vi "Plot Data - Configure Plot GUI.vi"(8 "Error In":errorcluster, 11 "Plot Channel Configurations In":T1[](array[typedef])) -> (0 "Error Out":errorcluster, 3 "Plot Channel Configurations Out":T1[](array[typedef]))   [LabVIEW 2017, in "DTacq Plot Display Library.lvlib"]
uses:
  DTacq Plot Display Library.lvlib
  Typedefs/Plot Channel Configruation--Cluster.ctl
  Typedefs/Graphical Interface Commands - Configuration--Enum.ctl
  Network Shared Variables/Typedefs/Shared Variable Properties--Cluster.ctl
  Network Shared Variables/Shared Variables Library.lvlib
panel:
  in  "Paste Button":bool
  in  "Cancel Button":bool
  in  "OK Button":bool
  in  "Plot Colour Box":u32(colorbox)
  in  "Multicolumn Listbox":i32(listbox)
  in  "Descriptive Name":string
  in  "Data Source Dropdown":u16(ring) items=["Carrier1Module1-ACQ425ELF-Channel_01", "Carrier1Module1-ACQ425ELF-Channel_02", "Carrier1Module1-ACQ425ELF-Channel_03", "Carrier1Module1-ACQ425ELF-Channel_04", "Carrier1Module1-ACQ425ELF-Channel_05", "Carrier1Module1-ACQ425ELF-Channel_06", "Carrier1Module1-ACQ425ELF-Channel_07", "Carrier1Module1-ACQ425ELF-Channel_08", "Carrier1Module1-ACQ425ELF-Channel_09", "Carrier1Module1-ACQ425ELF-Channel_10", "Carrier1Module1-ACQ425ELF-Channel_11", "Carrier1Module1-ACQ425ELF-Channel_12", "Carrier1Module1-ACQ425ELF-Channel_13", "Carrier1Module1-ACQ425ELF-Channel_14", "Carrier1Module1-ACQ425ELF-Channel_15", "Carrier1Module1-ACQ425ELF-Channel_16"]
  in  "Remove Button":bool
  in  "Add Button":bool
  # "Data Sources"
  # "Data Source"
  # "Name"
  # "Colour"
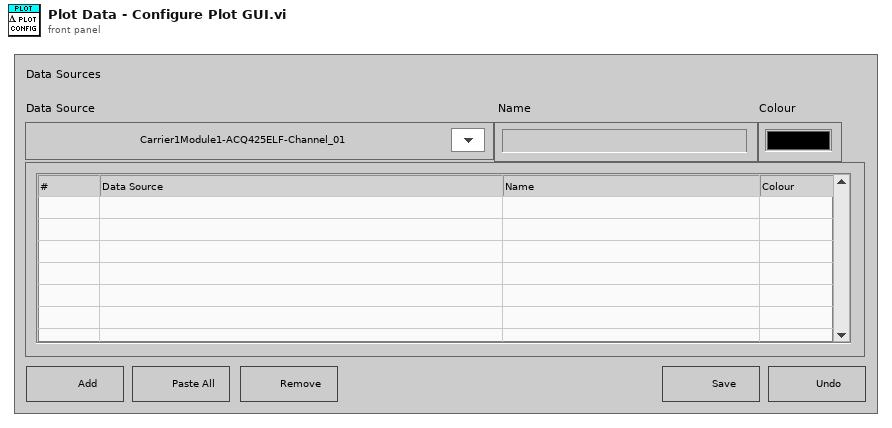
[diagram p1: front panel]
types:
  T1 = typedef "DTacq Plot Display Library.lvlib/Plot Channel Configruation--Cluster.ctl" = cluster{"Shared Variable Reference":refnum<k21>, "Full Variable Name":string, "URL":string, "Descriptive Name":string, "Data Type":variant, "Colour":u32}
  T2 = typedef "Shared Variables Library.lvlib/Shared Variable Properties--Cluster.ctl" = cluster{"Name":string, "URL":string, "Data Type":variant}
  T3 = typedef "DTacq Plot Display Library.lvlib/Graphical Interface Commands - Configuration--Enum.ctl" = enum16{"Cancel and Close", "Paste All", "Restore Previous", "Poll GUI", "Cancel", "Save", "Remove Channel", "Add Channel", "Initialise"}
  T4 = enum32{"Invalid", "Standard", "Closed", "Hidden", "Minimized", "Maximized"}
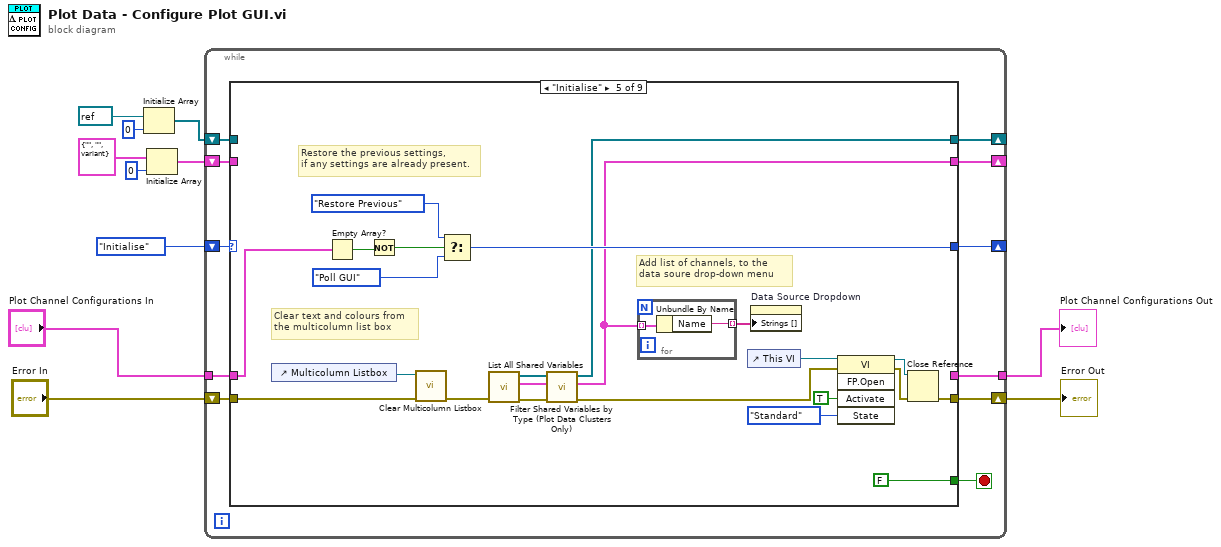
[diagram p0: block diagram]
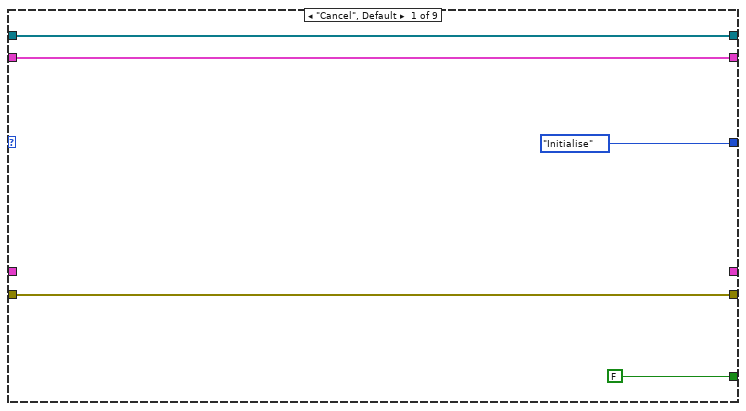
[diagram p2: hidden frame]
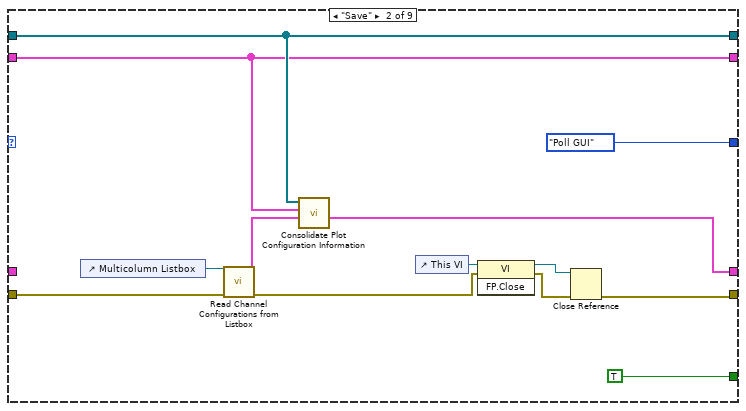
[diagram p3: hidden frame]
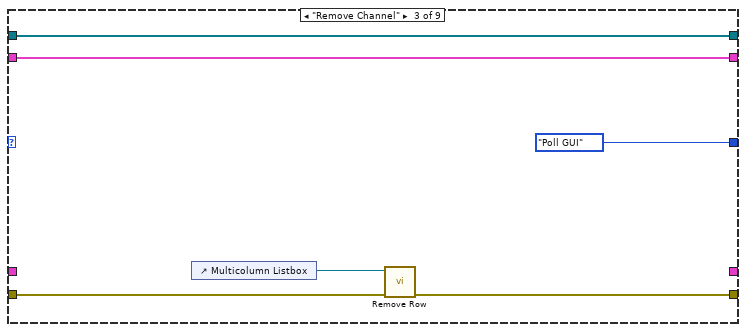
[diagram p4: hidden frame]
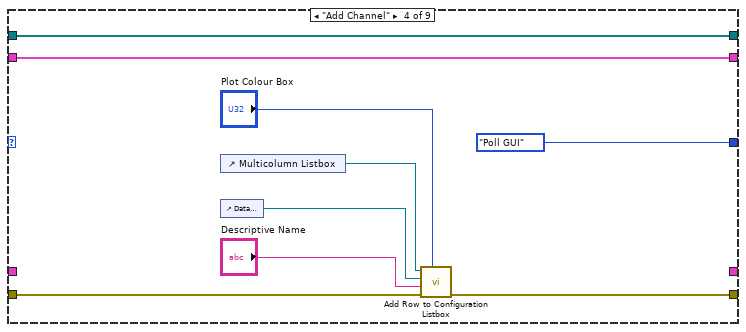
[diagram p5: hidden frame]
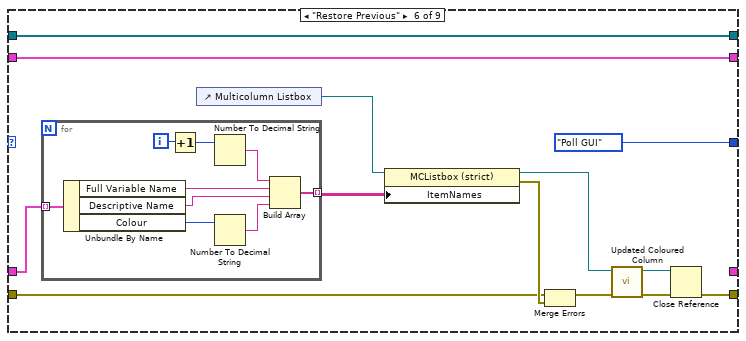
[diagram p6: hidden frame]
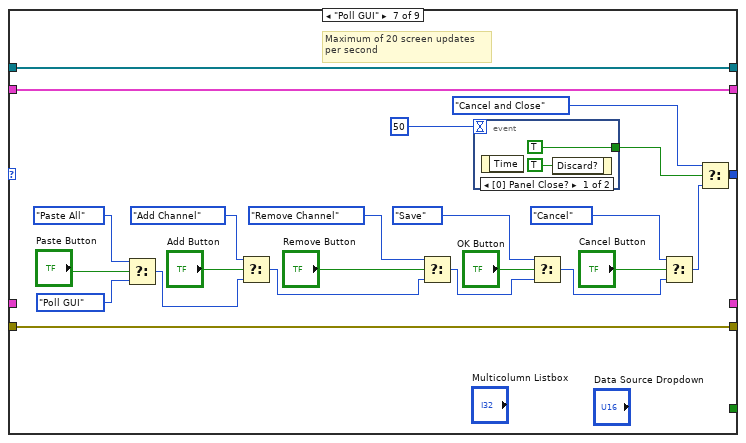
[diagram p7: hidden frame]
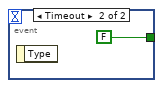
[diagram p8: hidden frame]
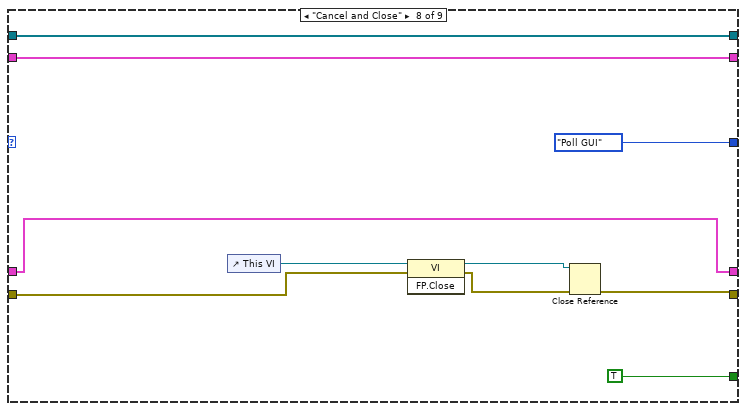
[diagram p9: hidden frame]
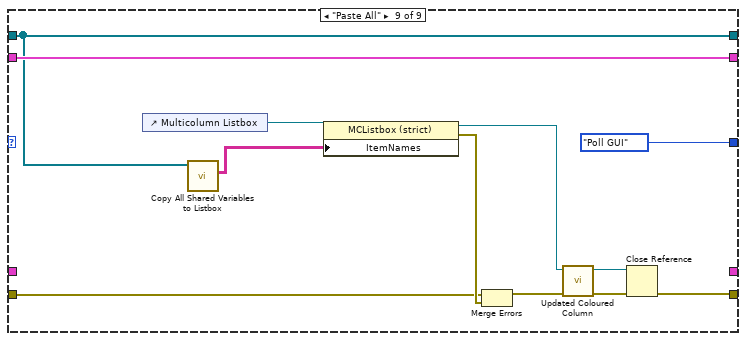
[diagram p10: hidden frame]
diagram:
  n1 = Initialize Array(refnum<k21> refnum, 0 ("dimension size")) -> (w8:refnum<k21>[])
  n2 = Initialize Array(T2 {"Name"="", "URL"="", "Data Type"=variant} ("Shared Variable Data"), 0 ("dimension size")) -> (w5:T2[])
  n3 = while {
    shift-right: [w20] -> w1
    shift-left: "Error In" -> [w21]
    shift-right: [w18] -> _
    shift-left: Graphical_Interface_Commands_-_Configuration--Enum."Initialise" -> [w22]
    shift-right: [w17] -> _
    shift-left: w8 -> [w16]
    shift-right: [w15] -> _
    shift-left: w5 -> [w14]
    tunnel: [w13] -> w4
    tunnel: "Plot Channel Configurations In" -> [w12]
    stop <- w19 stop-if-true
    n4 = case shown="\"Initialise\"" w22 {
      tunnel: w21 -> [w23 w35 w44 w54 w75 w85 w125 w135 w144]
      tunnel: [w23 w28 w43 w49 w70 w87 w125 w134 w140] -> w20
      tunnel: [FALSE TRUE _ _ FALSE _ _ TRUE _] -> w19
      tunnel: [Graphical_Interface_Commands_-_Configuration--Enum."Initialise" Graphical_Interface_Commands_-_Configuration--Enum."Poll GUI" Graphical_Interface_Commands_-_Configuration--Enum."Poll GUI" Graphical_Interface_Commands_-_Configuration--Enum."Poll GUI" w62 Graphical_Interface_Commands_-_Configuration--Enum."Poll GUI" w106 Graphical_Interface_Commands_-_Configuration--Enum."Poll GUI" Graphical_Interface_Commands_-_Configuration--Enum."Poll GUI"] -> w18
      tunnel: [w26 w38 w42 w48 w56 w93 w113 w138 w148] -> w17
      tunnel: w16 -> [w26 w38 w42 w48 _ w93 w113 w138 w148]
      tunnel: [w25 w37 w41 w47 w57 w92 w112 w137 w150] -> w15
      tunnel: w14 -> [w25 w37 w41 w47 _ w92 w112 w137 w150]
      tunnel: [_ w34 _ _ _ _ _ w133 _] -> w13
      tunnel: w12 -> [_ _ _ _ w67 w89 _ w133 _]
      frame "Cancel", Default {
      }
      frame "Save" {
        n5 = control-ref of="Multicolumn Listbox"() -> (w39:refnum<vi>)
        n6 = call "Read Channel Configurations from Listbox.vi"("error in"=w35, "MulticolumnListbox in"=w39) -> ("error out"=w29:errorcluster, "Plot Channel Configurations"=w36:T1[])  [unwired: 8 in]
        n7 = call "Consolidate Plot Configuration Information.vi"("Plot Channel Configurations"=w36, "Variable Descriptions"=w37, "Variable References"=w38) -> ("Plot Channel Configurations"=w34:T1[])  [unwired: 8 in]
        n8 = control-ref of="This VI"() -> (w32:refnum<vi>)
        n9 = invoke class="VI" method="FP.Close"(reference=w32, error in=w29) -> (reference out=w31:refnum<vi>, error out=w30:errorcluster)  [unwired: 1 in, 1 out]
        n10 = Close Reference(reference=w31, error in (no error)=w30) -> (error out=w28:errorcluster)
      }
      frame "Remove Channel" {
        n11 = control-ref of="Multicolumn Listbox"() -> (w45:refnum<vi>)
        n12 = call "Remove Row.vi"("error in"=w44, "MulticolumnListbox in"=w45) -> ("error out"=w43:errorcluster)  [unwired: 9 in]
      }
      frame "Add Channel" {
        n13 = control-ref of="Multicolumn Listbox"() -> (w53:refnum<vi>)
        n14 = control-ref of="Data Source Dropdown"() -> (w52:refnum<vi>)
        n15 = call "Add Row to Configuration Listbox.vi"("Plot Colour Box"="Plot Colour Box", "error in"=w54, "Descriptive Name"="Descriptive Name", "Data Source Selector Ref"=w52, "Configuraiton Listbox Ref"=w53) -> ("error out"=w49:errorcluster)  [unwired: 6 in]
      }
      frame "Initialise" {
        # "Restore the previous settings,\nif any settings are already present."
        # "Add list of channels, to the\ndata soure drop-down menu"
        # "Clear text and colours from\nthe multicolumn list box"
        n16 = control-ref of="Multicolumn Listbox"() -> (w76:refnum<vi>)
        n17 = Empty Array?(array=w67) -> (empty?=w66:bool)
        n18 = Not(x=w66) -> (.not. x?=w65:bool)
        n19 = call "Clear Multicolumn Listbox.vi"("error in"=w75, "MulticolumnListbox in"=w76) -> ("error out"=w74:errorcluster)  [unwired: 9 in]
        n20 = Select(t=Graphical_Interface_Commands_-_Configuration--Enum."Restore Previous", s=w65, f=Graphical_Interface_Commands_-_Configuration--Enum."Poll GUI") -> (s? t:f=w62:T3)
        n21 = call "List All Shared Variables.vi"("error in"=w74) -> ("error out"=w59:errorcluster, "Variable Descriptions"=w60:T2[], "Variable References"=w61:refnum<k21>[])  [unwired: 8 in]
        n22 = call "Filter Shared Variables by Type (Plot Data Clusters Only).vi"("error in"=w59, "Variable Descriptions"=w60, "Variable References"=w61) -> ("error out"=w58:errorcluster, "Variable Descriptions"=w57:T2[], "Shared Variable References"=w56:refnum<k21>[])  [unwired: 6 in]
        n23 = for {
          tunnel: w57 -> [w80] mode=indexing
          tunnel: [w79] -> w78 mode=indexing
          n24 = Unbundle By Name(w80) -> ("Name"=w79:string)
        }
        n25 = control-ref of="This VI"() -> (w73:refnum<vi>)
        n26 = property on="Data Source Dropdown" class="Ring (strict)"("Strings []"=w78) -> ()  [unwired: 2 in, 2 out]
        n27 = invoke class="VI" method="FP.Open"(reference=w73, error in=w58, "Activate"=TRUE ("Activate?"), "State"=T4."Standard") -> (reference out=w69:refnum<vi>, error out=w68:errorcluster)  [unwired: 1 in, 3 out]
        n28 = Close Reference(reference=w69, error in (no error)=w68) -> (error out=w70:errorcluster)
      }
      frame "Restore Previous" {
        n29 = for {
          tunnel: w89 -> [w102] mode=indexing
          tunnel: [w96] -> w88 mode=indexing
          i -> [w95]
          n30 = Unbundle By Name(w102) -> ("Full Variable Name"=w99:string, "Descriptive Name"=w98:string, "Colour"=w101:u32)
          n31 = Increment(x=w95) -> (x+1=w94:i32)
          n32 = Number To Decimal String(number=w94) -> (decimal integer string=w100:string)  [unwired: 1 in]
          n33 = Number To Decimal String(number=w101) -> (decimal integer string=w97:string)  [unwired: 1 in]
          n34 = Build Array(w100, w99, w98, w97) -> (w96:string[])
        }
        n35 = control-ref of="Multicolumn Listbox"() -> (w90:refnum<vi>)
        n36 = property class="MCListbox (strict)"(reference=w90, "ItemNames"=w88) -> (reference out=w81:refnum<vi>, error out=w86:errorcluster)  [unwired: 1 in]
        n37 = Merge Errors(w85, w86) -> (w82:errorcluster)
        n38 = call "Updated Coloured Column.vi"("error in"=w82, "MulticolumnListbox in"=w81) -> ("error out"=w83:errorcluster, "MulticolumnListbox Out"=w84:refnum<vi>)  [unwired: 8 in]
        n39 = Close Reference(reference=w84, error in (no error)=w83) -> (error out=w87:errorcluster)
      }
      frame "Poll GUI" {
        # "Maximum of 20 screen updates\nper second"
        n40 = Select(t=Graphical_Interface_Commands_-_Configuration--Enum."Paste All", s="Paste Button", f=Graphical_Interface_Commands_-_Configuration--Enum."Poll GUI") -> (s? t:f=w104:T3)
        n41 = Select(t=Graphical_Interface_Commands_-_Configuration--Enum."Add Channel", s="Add Button", f=w104) -> (s? t:f=w117:T3)
        n42 = Select(t=Graphical_Interface_Commands_-_Configuration--Enum."Remove Channel", s="Remove Button", f=w117) -> (s? t:f=w119:T3)
        n43 = event shown="[0] Panel Close?" {
          selector: _ -> [_ _]
          dyn-events: _ -> [_ _]
          timeout: u32 50 ("milliseconds to wait") -> [_ _]
          tunnel: [TRUE ("Discard?") FALSE] -> w108
          event Panel Close? {
            n44 = event-data() -> ()  [unwired: 1 in, 1 out]
            n45 = event-data("Discard?"=TRUE) -> ()  [unwired: 1 in, 1 out]
          }
          event Timeout {
            n46 = event-data() -> ()  [unwired: 1 in, 1 out]
          }
        }
        n47 = Select(t=Graphical_Interface_Commands_-_Configuration--Enum."Save", s="OK Button", f=w119) -> (s? t:f=w114:T3)
        n48 = Select(t=Graphical_Interface_Commands_-_Configuration--Enum."Cancel", s="Cancel Button", f=w114) -> (s? t:f=w105:T3)
        n49 = Select(t=Graphical_Interface_Commands_-_Configuration--Enum."Cancel and Close", s=w108, f=w105) -> (s? t:f=w106:T3)
      }
      frame "Cancel and Close" {
        n50 = control-ref of="This VI"() -> (w136:refnum<vi>)
        n51 = invoke class="VI" method="FP.Close"(reference=w136, error in=w135) -> (reference out=w130:refnum<vi>, error out=w131:errorcluster)  [unwired: 1 in, 1 out]
        n52 = Close Reference(reference=w130, error in (no error)=w131) -> (error out=w134:errorcluster)
      }
      frame "Paste All" {
        n53 = control-ref of="Multicolumn Listbox"() -> (w149:refnum<vi>)
        n54 = call "Copy All Shared Variables to Listbox.vi"("Array"=w148) -> ("Listbox Data"=w147:string[][])  [unwired: 10 in]
        n55 = property class="MCListbox (strict)"(reference=w149, "ItemNames"=w147) -> (reference out=w146:refnum<vi>, error out=w145:errorcluster)  [unwired: 1 in]
        n56 = Merge Errors(w144, w145) -> (w143:errorcluster)
        n57 = call "Updated Coloured Column.vi"("error in"=w143, "MulticolumnListbox in"=w146) -> ("error out"=w142:errorcluster, "MulticolumnListbox Out"=w141:refnum<vi>)  [unwired: 8 in]
        n58 = Close Reference(reference=w141, error in (no error)=w142) -> (error out=w140:errorcluster)
      }
    }
  }
  "Plot Channel Configurations Out" <- w4
  "Error Out" <- w1
